vi "Get Buffer.vi"(8 "error in (no error)":errorcluster, 11 "Carya Config in":refnum<class "Carya Config (By Reference).lvclass">) -> (0 "error out":errorcluster, 3 "Config":refnum<class "Carya Config (By Reference).lvclass">)   [LabVIEW 2013, in "Carya Config (By Reference).lvclass"]
doc: "Copyright 2018, Carya Automatisering, Wiebe Walstra."
uses:
  Carya Config (By Reference).lvclass
  Carya Config (By Reference).lvclass/Carya Config (By Reference).ctl
  CConfig Buffer Type/CConfig Buffer Type.lvclass
  Carya Config.lvclass
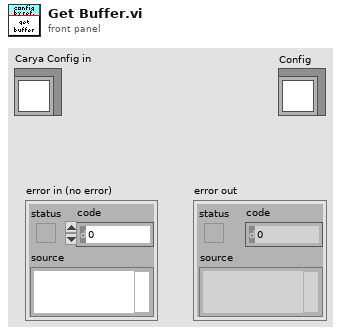
[diagram p1: front panel]
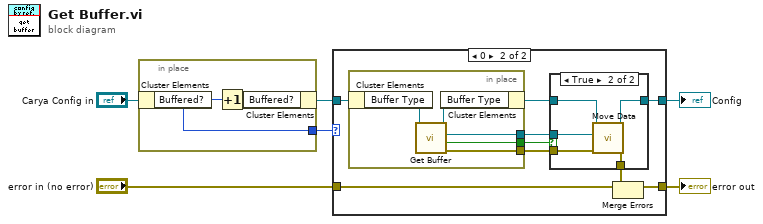
[diagram p0: block diagram]
diagram:
  n1 = in-place {
    in-place-border: [w7] -> w1
    n2 = in-place-cluster #1("Carya Config in") -> ("Buffered?"=w7:i32)
    n3 = Increment(x=w7) -> (x+1=w8:i32)
    n4 = in-place-cluster #1("Buffered?"=w8) -> (w2:refnum<class "Carya Config (By Reference).lvclass">)
  }
  n5 = case shown="0" w1 {
    tunnel: [w9 w19] -> w6
    tunnel: "error in (no error)" -> [w9 w18]
    tunnel: [w10 w14] -> w4
    tunnel: w2 -> [w10 w13]
    frame Default {
    }
    frame 0 {
      n6 = in-place {
        in-place-border: [w31] -> w17
        in-place-border: [w30] -> w16
        in-place-border: [w27] -> w11
        n7 = in-place-cluster #2(w13) -> ("Buffer Type"=w29:refnum<class "CConfig Buffer Type.lvclass">)
        n8 = call-dynamic "Get Buffer.vi"("CConfig Buffer Type"=w29) -> ("error out"=w30:errorcluster, "Copy data?"=w27:bool, "Config"=w31:refnum<class "Carya Config.lvclass">, "CConfig Buffer Type"=w28:refnum<class "CConfig Buffer Type.lvclass">)  [unwired: 7 in]
        n9 = in-place-cluster #2("Buffer Type"=w28) -> (w12:refnum<class "Carya Config (By Reference).lvclass">)
      }
      n10 = case shown="True" w11 {
        tunnel: w17 -> [_ w26]
        tunnel: w16 -> [w20 w25]
        tunnel: [w20 w24] -> w15
        tunnel: [w21 w23] -> w14
        tunnel: w12 -> [w21 w22]
        frame False {
        }
        frame True {
          n11 = call "Move Data.vi"("error in (no error)"=w25, "Carya Config source"=w26, "Carya Config dest"=w22) -> ("error out"=w24:errorcluster, "Carya Config out"=w23:refnum<class "Carya Config (By Reference).lvclass">)  [unwired: 7 in]
        }
      }
      n12 = Merge Errors(w18, w15) -> (w19:errorcluster)
    }
  }
  "error out" <- w6
  "Config" <- w4
